vi "Create Interpolating Polynomial.vi"(10 "coefficients":dbl[][](array[numeric]) format="%.4g", 11 "x locations":dbl[](array[numeric]) format="%.4g") -> (0 "error":i32, 3 "piecewise polynomial":T1 {"x locations" format="%.4g"; "coefficients" format="%.4g"})   [LabVIEW 2017, in "NI_Gmath.lvlib"]
doc: "Takes the piecewise polynomial <B>x locations</B> and a 2D array of <B>coefficients</B> and forms the <B>piecewise polynomial</B> cluster for the Evaluate Interpolating Polynomial VI to use."
uses:
  NI_Gmath.lvlib
  in_piecewise interp poly control.ctl
panel:
  # "Create Interpolating Polynomial"
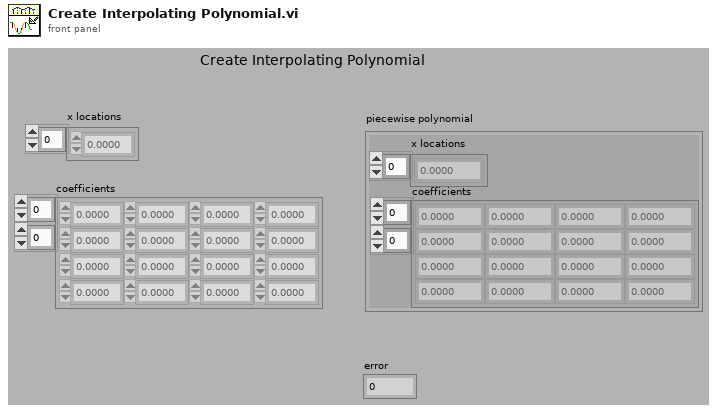
[diagram p1: front panel]
types:
  T1 = typedef "NI_Gmath.lvlib/in_piecewise interp poly control.ctl" = cluster{"x locations":dbl[], "coefficients":dbl[][]}
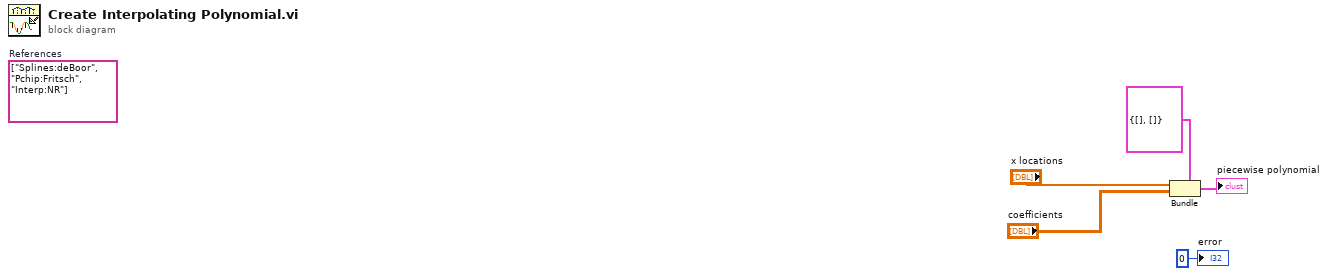
[diagram p0: block diagram]
diagram:
  (unwired) string[] ["Splines:deBoor", "Pchip:Fritsch", "Interp:NR"]  # References
  n1 = Bundle(cluster=T1 {"x locations"=[], "coefficients"=[]} ("piecewise polynomial"), "x locations"="x locations", "coefficients"="coefficients") -> (→"piecewise polynomial":T1)
  "error" <- 0 ("error")
